vi "User_Input_Demo.vi"   [LabVIEW 2017, in "Examples.lvlib"]
uses:
  Examples.lvlib
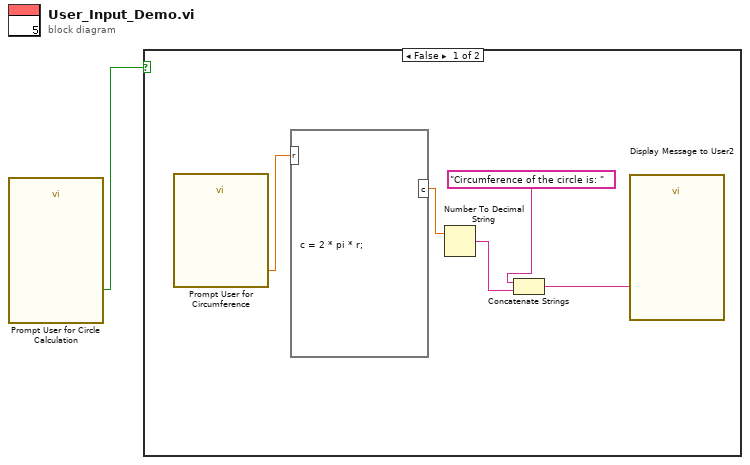
[diagram p0: block diagram]
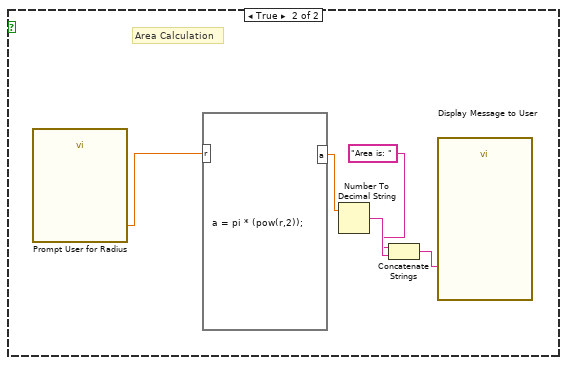
[diagram p2: hidden frame]
diagram:
  n1 = call "Prompt User for Circle Calculation"() -> ("Area"=w1:bool)  [unwired: 16 in, 3 out]
  n2 = case shown="False" w1 {
    frame False {
      n3 = call "Prompt User for Circumference"() -> ("circumference"=w6:dbl)  [unwired: 17 in, 2 out]
      n4 = formula code="c = 2 * pi * r;"("r"=w6) -> ("c"=w5:dbl)
      n5 = Number To Decimal String(number=w5) -> (decimal integer string=w4:string)  [unwired: 1 in]
      n6 = Concatenate Strings("Circumference of the circle is: ", w4) -> (w2:string)
      n7 = call "Display Message to User2"("Message"=w2) -> ()  [unwired: 9 in, 2 out]
    }
    frame True {
      # "Area Calculation"
      n8 = call "Prompt User for Radius"() -> ("radius"=w11:dbl)  [unwired: 17 in, 2 out]
      n9 = formula code="a = pi * (pow(r,2));"("r"=w11) -> ("a"=w10:dbl)
      n10 = Number To Decimal String(number=w10) -> (decimal integer string=w8:string)  [unwired: 1 in]
      n11 = Concatenate Strings("Area is: ", w8) -> (w9:string)
      n12 = call "Display Message to User"("Message"=w9) -> ()  [unwired: 9 in, 2 out]
    }
  }
